vi "ILD_15%.vi"(5 "Frequency(Hz)":dbl[](array[numeric]), 6 "specData":string[][](array[string]), 7 "2x":dbl[](array[numeric]), 8 "ILD data":dbl[][](array[numeric]), 9 "2x equalize":bool) -> (0 "ILD_15% result":bool[](array[boolean]), 1 "ILD_15ChartData":T1(array[cluster]), 2 "ILD_15%":dbl[](array[numeric]))   [LabVIEW 2011]
uses:
  <vilib>/measure/mamon.llb/Limit Testing Time.vi
  <vilib>/measure/NI_MAPro.lvlib
panel:
  out "转置的数组":dbl[][](array[numeric])
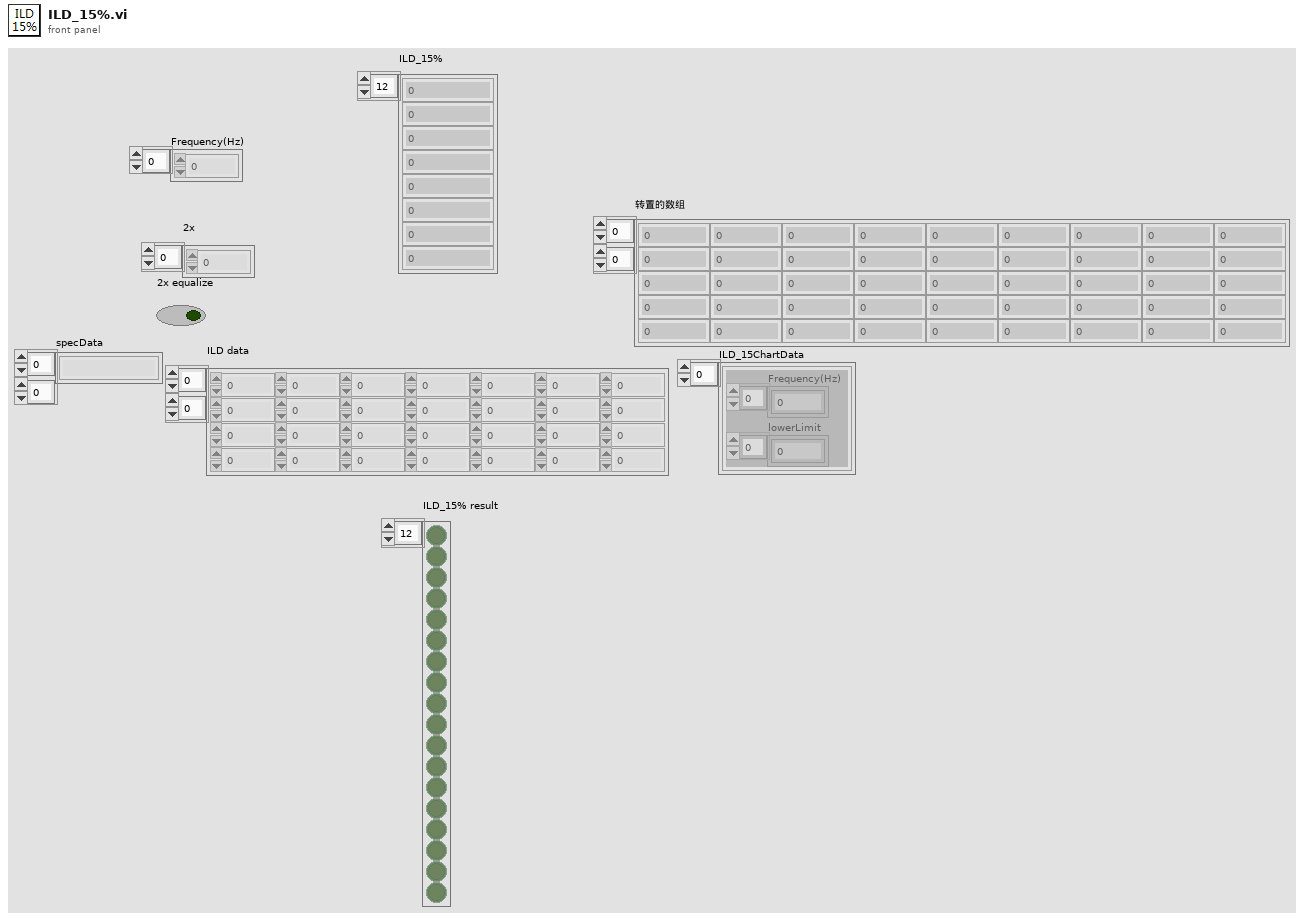
[diagram p1: front panel]
types:
  T1 = cluster{"Frequency(Hz)":dbl[], "lowerLimit":dbl[]}[]
  T2 = cluster{"Frequency(Hz)":dbl[], "lowerLimit":dbl[]}
  T3 = cluster{"Frequency(Hz)":dbl[], "upperLimit":dbl[]}
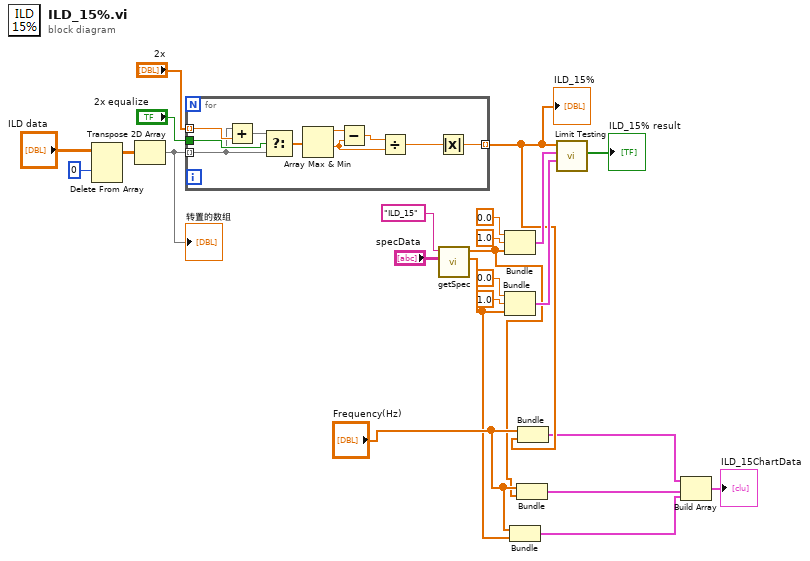
[diagram p0: block diagram]
diagram:
  n1 = Delete From Array(array="ILD data", index (row)=0 ("索引 (行)")) -> (array with subset deleted=w22:dbl[][])  [unwired: 2 in, 1 out]
  n2 = Transpose 2D Array(2D array=w22) -> (transposed array=w21:dbl[][])
  "转置的数组" <- w21
  n3 = for {
    tunnel: w21 -> [w24] mode=indexing
    tunnel: [w30] -> w8 mode=indexing
    tunnel: "2x" -> [w27] mode=indexing
    tunnel: "2x equalize" -> [w28]
    n4 = Add(x=w24, y=w27) -> (x+y=w26:dbl[])
    n5 = Select(t=w26, s=w28, f=w24) -> (s? t:f=w25:dbl[])
    n6 = Array Max & Min(array=w25) -> (max value=w32:dbl, min value=w29:dbl)  [unwired: 2 out]
    n7 = Subtract(x=w32, y=w29) -> (x-y=w33:dbl)
    n8 = Divide(x=w33, y=w29) -> (x/y=w31:dbl)
    n9 = Absolute Value(x=w31) -> (abs(x)=w30:dbl)
  }
  "ILD_15%" <- w8
  n10 = call "getSpec.vi"("specData"="specData", "itemName"="ILD_15") -> ("lowerLimit"=w5:dbl[], "upperLimit"=w6:dbl[])  [unwired: 8 in]
  n11 = Bundle(0.0, 1.0, "upperLimit"=w6) -> (w11:cluster{dbl, dbl, "upperLimit":dbl[]})  [unwired: 1 in]
  n12 = Bundle(0.0, 1.0, "lowerLimit"=w5) -> (w10:cluster{dbl, dbl, "lowerLimit":dbl[]})  [unwired: 1 in]
  n13 = Bundle("Frequency(Hz)"="Frequency(Hz)", "lowerLimit"=w5) -> (w2:T2)  [unwired: 1 in]
  n14 = Bundle("Frequency(Hz)"="Frequency(Hz)", "upperLimit"=w6) -> (w3:T3)  [unwired: 1 in]
  n15 = Bundle("Frequency(Hz)"="Frequency(Hz)", w8) -> (w4:cluster{"Frequency(Hz)":dbl[], dbl[]})  [unwired: 1 in]
  n16 = call-poly <vilib>:"Limit Testing.vi"("lower limit"=w10, "upper limit"=w11, "signal in"=w8) -> ("test results"=→"ILD_15% result":bool[])  [unwired: 3 in, 5 out]
  n17 = Build Array(w4, w3, w2) -> (→"ILD_15ChartData":T1)
